vi "Execute.GetProfilePath.vi"(8 "error in (no error)":errorcluster, 10 "base path":path, 11 "Profiles":refnum<vi>) -> (0 "error out":errorcluster, 3 "Path":path)   [LabVIEW 2013, in "Simple Sequence Tools - Execution.lvlib"]
uses:
  Simple Sequence Tools - Execution.lvlib
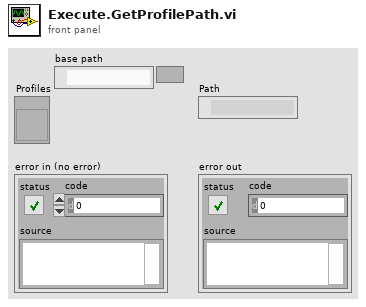
[diagram p1: front panel]
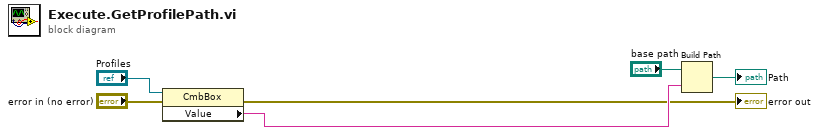
[diagram p0: block diagram]
diagram:
  n1 = property class="CmbBox"(reference="Profiles", error in="error in (no error)") -> (error out=→"error out":errorcluster, "Value"=w3:string)  [unwired: 1 out]
  n2 = Build Path(base path="base path", name or relative path=w3) -> (appended path=→"Path":path)
